vi "ServantTest.vi"() -> ()   [LabVIEW 2014]
panel:
  in  "input":dbl format="%#_13g"
  in  "Boolean":bool
  out "output":dbl format="%#_13g"
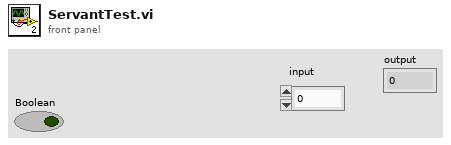
[diagram p1: front panel]
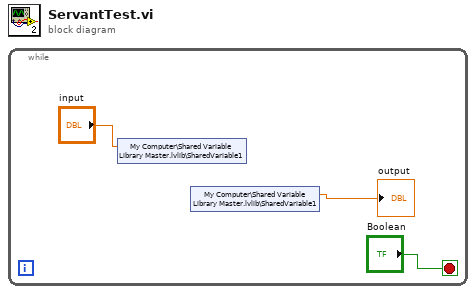
[diagram p0: block diagram]
diagram:
  n1 = while {
    stop <- "Boolean" stop-if-true
    n2 = shared-variable "My Computer\\Shared Variable Library Master.lvlib\\SharedVariable1"("input") -> ()  [unwired: 1 in, 1 out]
    n3 = shared-variable "My Computer\\Shared Variable Library Master.lvlib\\SharedVariable1"() -> (→"output":dbl)  [unwired: 1 in, 1 out]
  }
